vi "Wait Chart.vi"() -> ()   [LabVIEW 2022 SP3]
panel:
  out "Previous Iteration":dbl
  out "Top iteration":dbl
  out "Output":dbl
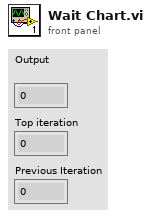
[diagram p1: front panel]
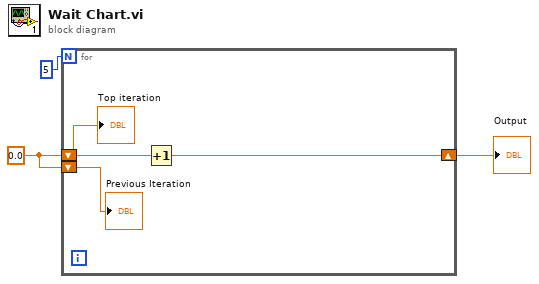
[diagram p0: block diagram]
diagram:
  w1 = 0.0
  n1 = for {
    N: 5 -> [_]
    shift-right: [w5] -> w2
    shift-left: w1 -> [w6]
    shift-left: w1 -> [w4]
    n2 = Increment(x=w6) -> (x+1=w5:dbl)
    "Top iteration" <- w6
    "Previous Iteration" <- w4
  }
  "Output" <- w2
